vi "MainsubPanel.vi"() -> ()   [LabVIEW 2014]
doc: "Main\nThis is the main VI, and call via subpanel the other VI\n\nYou can click on the control and the selection on the menu.\n\nTo return in main subpanel press ESC.\n\n\nNicola Bavarone Bytelabs.it"
uses:
  SubPanel/SubPanelModule.lvlib
  MSQ_MessageQueues/Enqueue Message (Single).vi
  <vilib>/rvi/interface/nirviMethod/nirviMethod.xnode
  <vilib>/FPGAPlugInAG/Dynamic/niLvFpga_Reset_Dynamic.vi
  <vilib>/FPGAPlugInAG/Dynamic/niLvFpga_StartFifo_Dynamic.vi
  <vilib>/rvi/errors/niLvFpgaMergeErrorWithErrorCode.vi
  <vilib>/FPGAPlugInAG/Dynamic/niLvFpga_ConfigureFifo_Dynamic.vi
  <vilib>/FPGAPlugInAG/Dynamic/niLvFpga_Run_Dynamic.vi
  <vilib>/rvi/interface/nirviReadWriteControl/nirviReadWriteControl.xnode
  <vilib>/rvi/interface/Simulation/niFpgaSimulationCallBeginRW.vi
  <vilib>/rvi/errors/niLvFpgaAdjustHostInterfaceError.vi
  <vilib>/FPGAPlugInAG/Dynamic/niLvFpga_WriteFifo_Dynamic.vi
  <vilib>/rvi/interface/nirviCloseFPGA/nirviCloseFPGA.xnode
  <vilib>/FPGAPlugInAG/Dynamic/niLvFpga_Close_Dynamic.vi
  <vilib>/rvi/interface/nirviOpenFPGA/nirviOpenFPGA.xnode
  FPGA Bitfiles/LaserWaveMatrix_FPGATarget_LaserWaveFPGA_x7ByfWROQXI.lvbitx
  Fpga/FpgaMain.vi
panel:
  in  "NEW STRING":string="INSERISCI QUI LA TUA STRINGA"
  out "AO FIFO Empty":bool
  out "Empty Elements Remaining":u32
  out "# Loop":i32=83
  in  "Ton (ticks)":u32=40
  in  "Toff (ticks)":u32=40
  out "Elem act":u8
  in  "PRINT":bool
  out "Date":string
  out "Time":string
  # "EXTREME FM-X121"
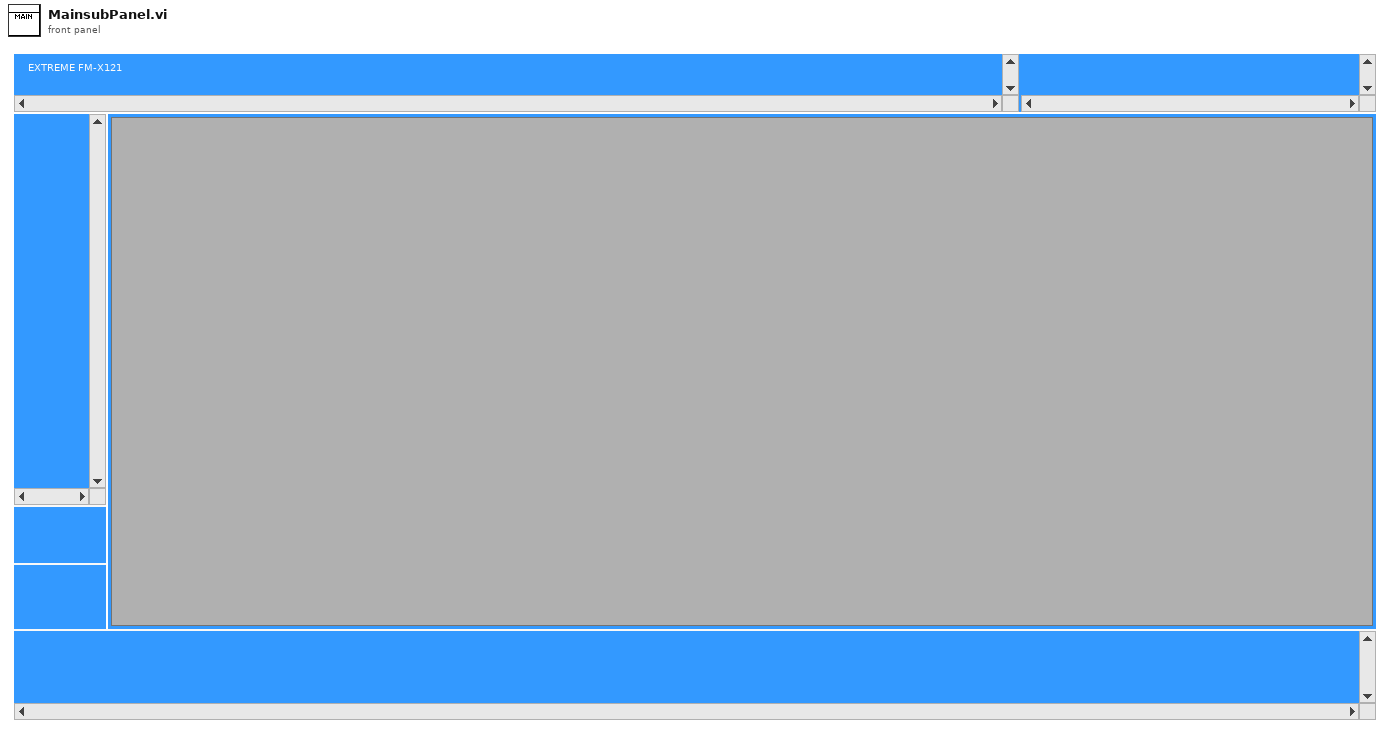
[diagram p1: front panel]
types:
  T1 = cluster{"Buffer_U64":u64[], "# Chart":i32, "BufferString":string[], "TotalStringBuff":i32, "over buffer":bool, "Ton (ticks)":u32, "Toff (ticks)":u32, "EmptyEl_Rem":u32}
  T2 = enum32{"invalid app kind", "Development System", "Run Time System", "Student Edition", "Embedded LabVIEW", "Evaluation", "Custom"}
  T3 = cluster{"UsrName":string, "UsrPsw":string, "UsrLevel":string}
  T4 = enum32{"Invalid", "Standard", "Closed", "Hidden", "Minimized", "Maximized"}
  T5 = typedef "eventvkey.ctl" = enum16{"ASCII", "Enter", "Return", "Shift", "Ctrl", "Alt", "Cmd", "Opt", "Caps", "NumLock", "Clear", "Break", "Up", "Down", "Left", "Right", "Insert", "Delete", "Home", "End", "PageUp", "PageDown", "Escape", "Help", "Pause", "ScrollLock", "F1", "F2", "F3", "F4", "F5", "F6", "F7", "F8", "F9", "F10", "F11", "F12", "F13", "F14", "F15", "F16", "F17", "F18", "F19", "F20", "F21", "F22", "F23", "F24", "Play", "VolumeUp", "VolumeDown", "Mute", "Two Byte Char"}
  T6 = enum32{"Bad", "Idle", "Run top level", "Running"}
  T7 = cluster{"Core":cluster{"Current VI Reference":refnum<vi>, "Close Panel on Exit?":bool}, "SubPanRefs":refnum<vi>[], "SubPanelsVis":string[], "SubP_VIsPathList":path[], "InsertedVIref":refnum<vi>, "Control Names":string[], "Values":variant[], "User":cluster{"UsrName":string, "UsrPsw":string, "UsrLevel":string}}
  T8 = cluster{"Current VI Reference":refnum<vi>, "Close Panel on Exit?":bool}
  T9 = typedef "Preset_Data.ctl" = cluster{"RS232config":T10, "USB_Config":T11, "PrintOffset":T12, "Aiming":T13, "Set Telnet TCPIP":T14}
  T10 = typedef "Rs232_Config.ctl" = cluster{"State":bool, "COM":string, "Baud Rate":i32, "Data Bit":i32, "Stop Bit":u16, "Parity":u16, "Flow Mode":u16}
  T11 = typedef "USB_Config.ctl" = cluster{"Status":bool, "COM":string}
  T12 = typedef "PrintOffset.ctl" = cluster{"PrintDelay":u32, "ForwardOffset":u32}
  T13 = typedef "Aiming.ctl" = cluster{"AimingBean":bool, "LaserTemperature":dbl, "SysTemperature":dbl}
  T14 = typedef "TCP_Config.ctl" = cluster{"State":bool, "IP ADDRESS":string, "Port":i32}
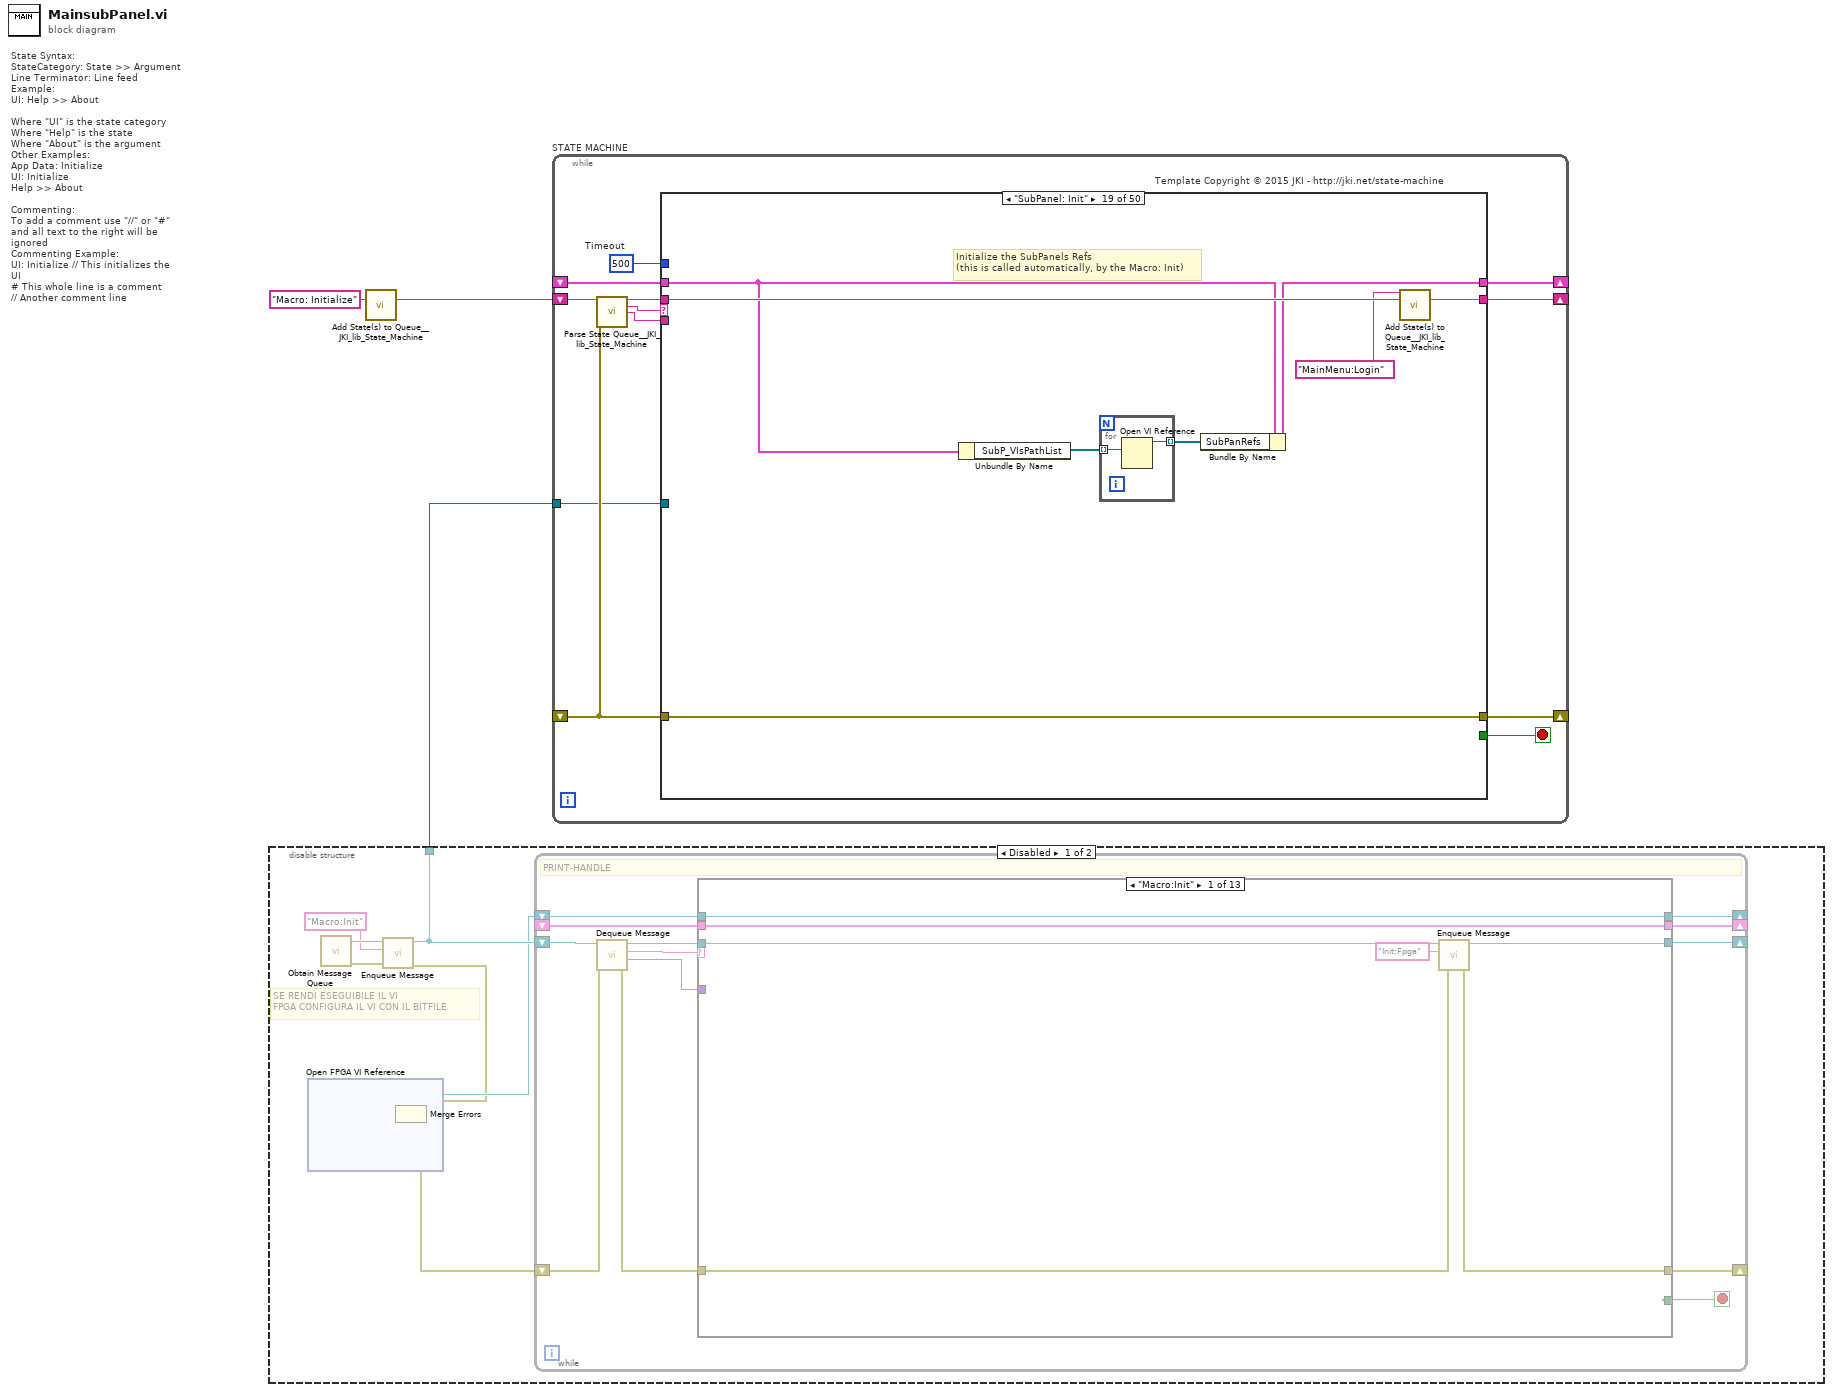
[diagram p0: block diagram]
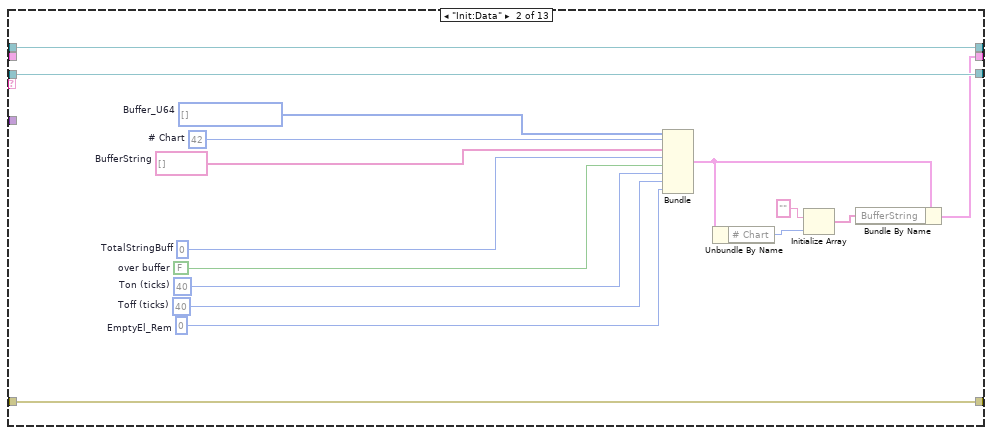
[diagram p2: hidden frame]
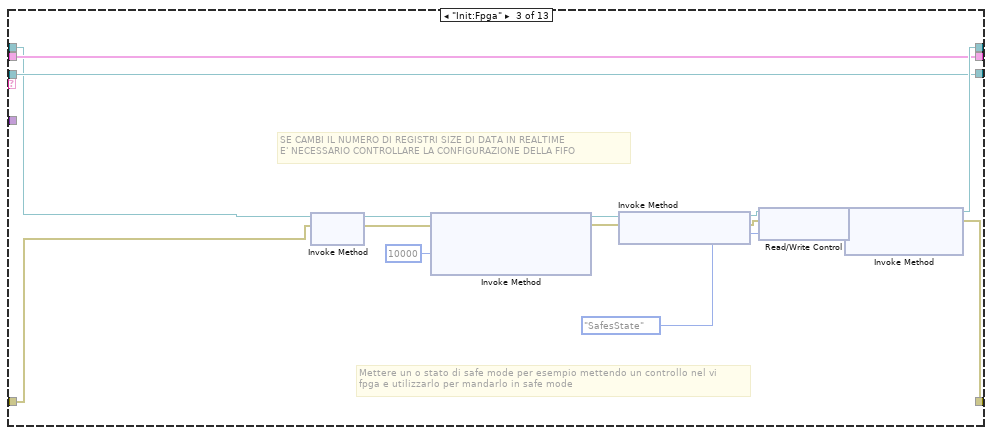
[diagram p3: hidden frame]
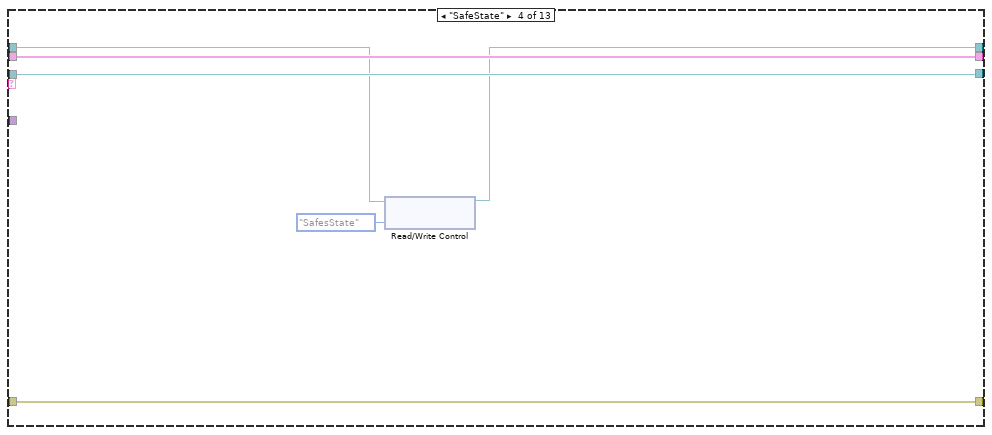
[diagram p4: hidden frame]
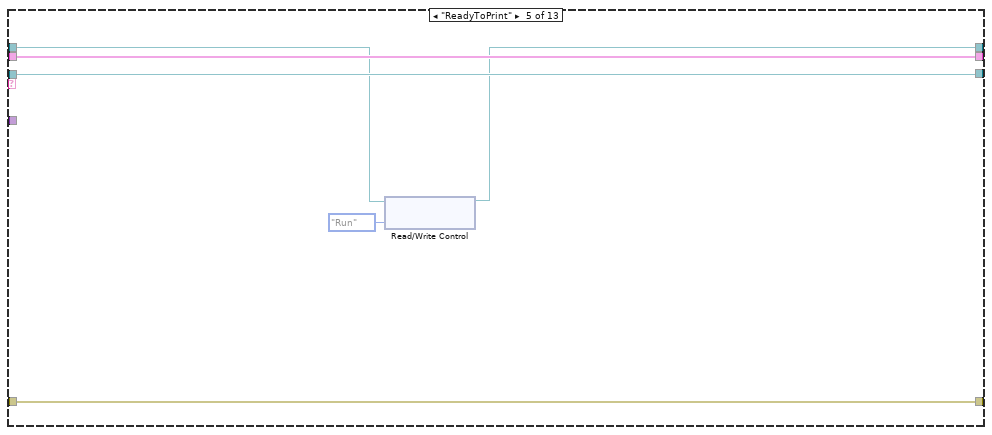
[diagram p5: hidden frame]
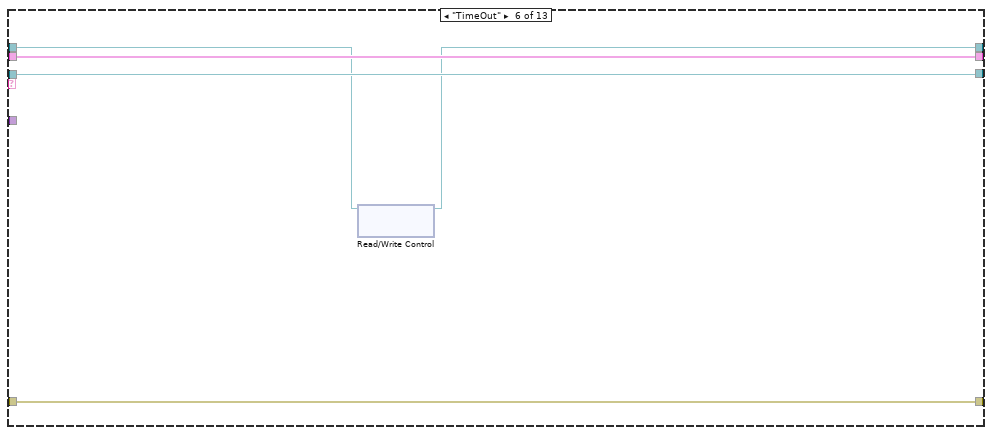
[diagram p6: hidden frame]
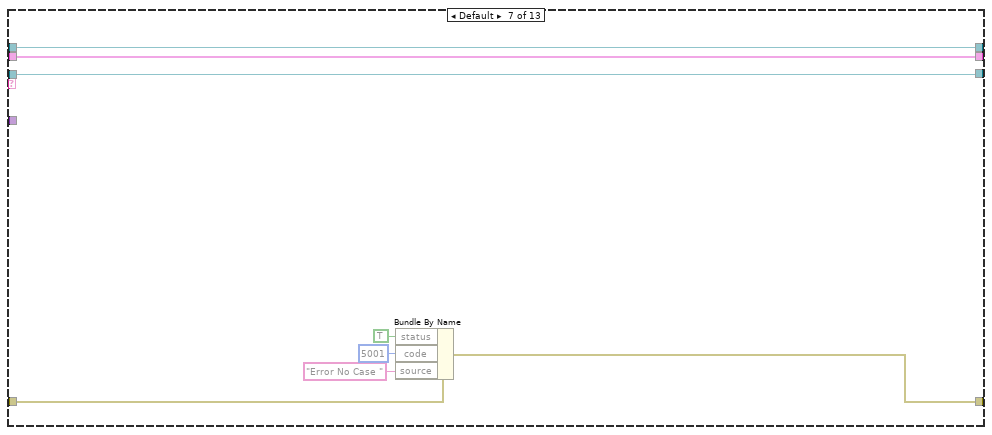
[diagram p7: hidden frame]
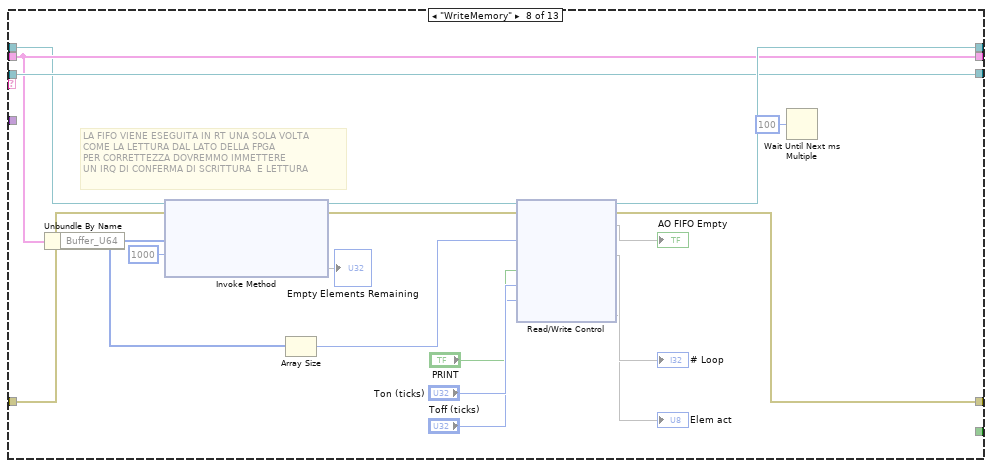
[diagram p8: hidden frame]
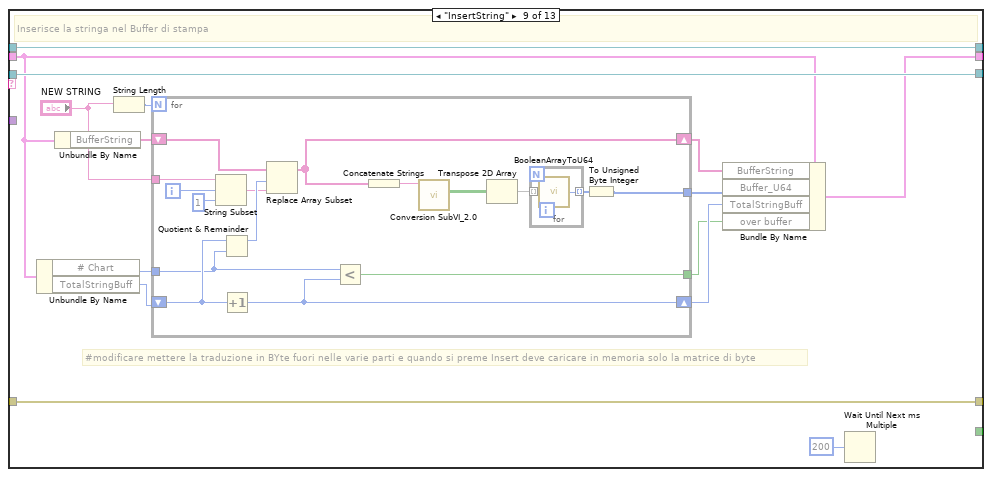
[diagram p9: hidden frame]
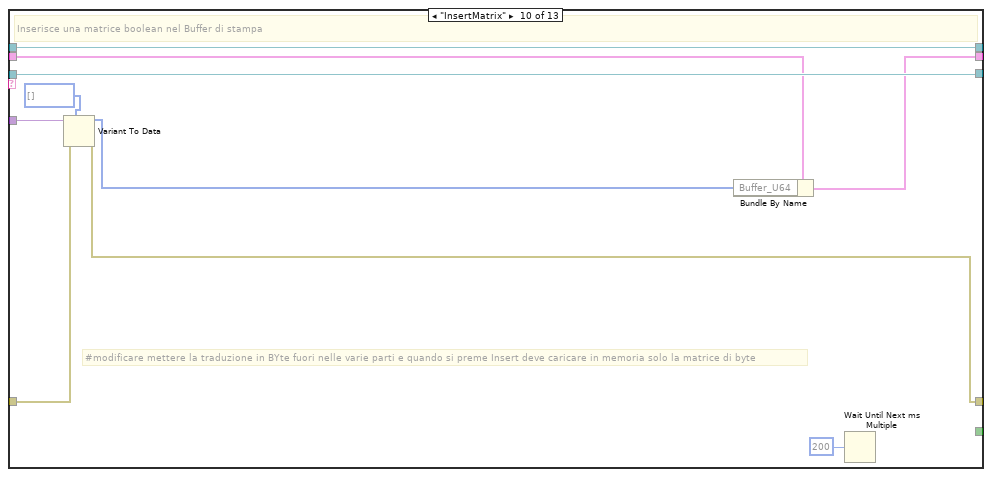
[diagram p10: hidden frame]
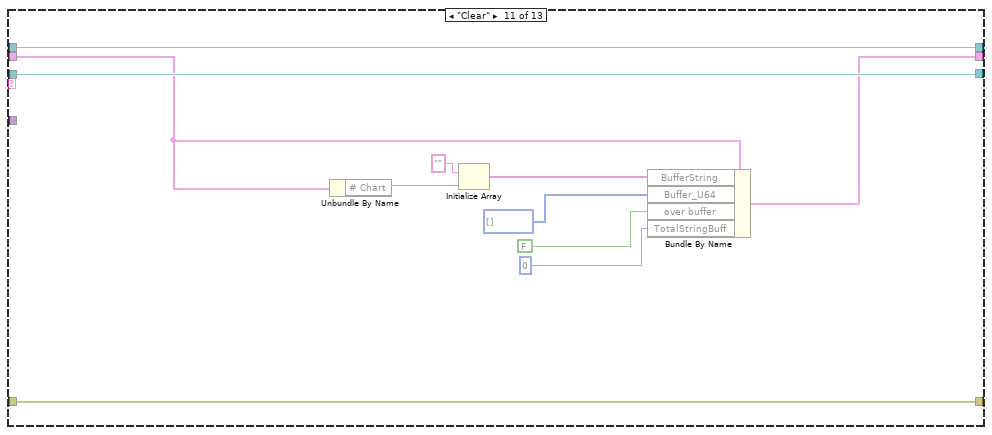
[diagram p11: hidden frame]
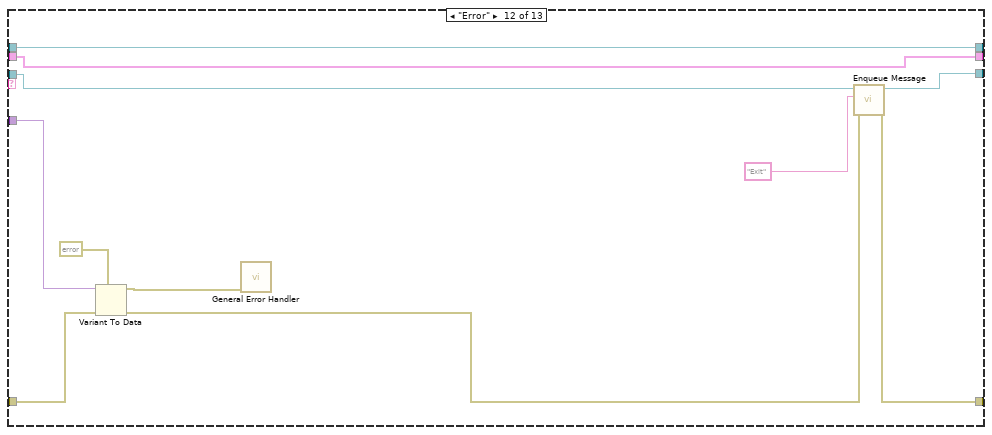
[diagram p12: hidden frame]
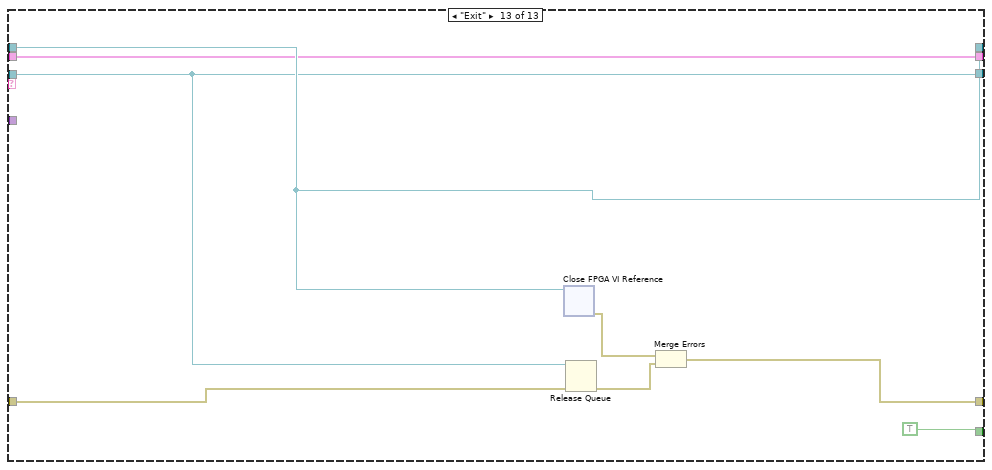
[diagram p13: hidden frame]
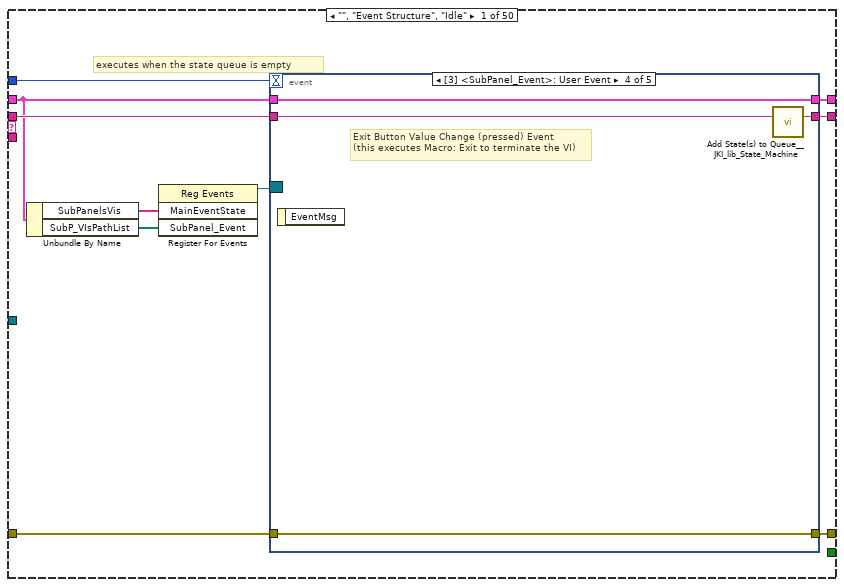
[diagram p15: hidden frame]
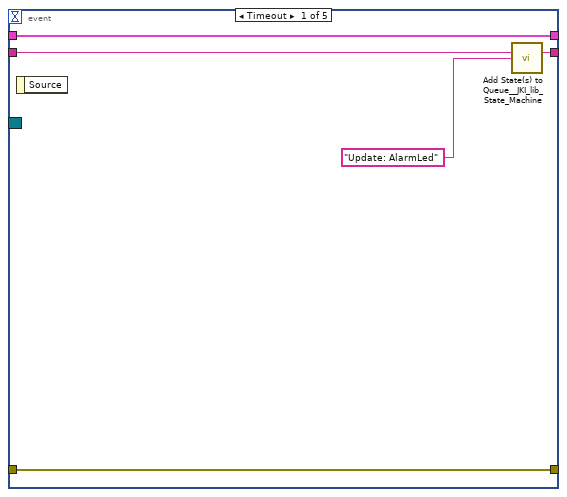
[diagram p16: hidden frame]
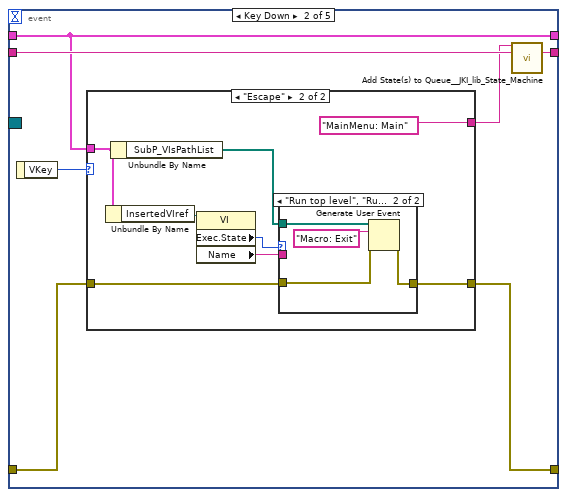
[diagram p17: hidden frame]
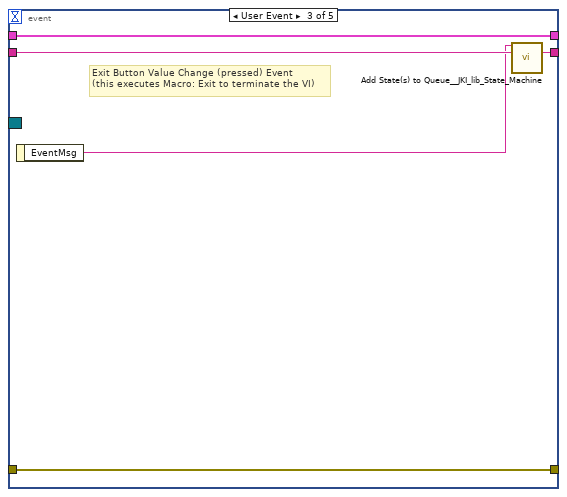
[diagram p20: hidden frame]
diagram:
  # "State Syntax:\nStateCategory: State >> Argument\nLine Terminator: Line feed\nExample:\nUI: Help >> About\n\nWhere \"UI\" is the state category\nWhere \"Help\" is the state\nWhere \"About\" is the argument\nOther Examples:\nApp Data: Initialize\nUI: Initialize\nHelp >> About\n\nCommenting:\nTo add a comment use \"//\" or \"#\" and all text to the right will be ignored\nCommenting Example:\nUI: Initialize // This initializes the UI\n# This whole line is a comment\n// Another comment line"
  n1 = disable-structure shown="Disabled" {
    disable-tunnel: [w8 _] -> w1
    frame Disabled {
      # "SE RENDI ESEGUIBILE IL VI \nFPGA CONFIGURA IL VI CON IL BITFILE"
      n2 = xnode "Open FPGA VI Reference"() -> ("FPGA VI Reference Out"=w7:refnum<k20>, "error out"=w6:errorcluster)  [unwired: 2 in]
      n3 = call "Obtain Message Queue.vi"() -> ("error out"=w10:errorcluster, "Message Queue"=w11:refnum<queue>)  [unwired: 10 in]
      n4 = call-poly "Enqueue Message.vi"("error in (no error)"=w10, "Message"="Macro:Init", "Message Queue"=w11) -> ("error out"=w4:errorcluster, "dup Message Queue"=w8:refnum<queue>)  [unwired: 7 in]
      n5 = Merge Errors(w4, w6) -> (w5:errorcluster)
      n6 = while {
        shift-right: [w22] -> _
        shift-left: w5 -> [w18]
        shift-right: [w23] -> _
        shift-left: w7 -> [w24]
        shift-right: [w20] -> _
        shift-left: w8 -> [w19]
        shift-right: [w12] -> _
        shift-left: _ -> [w13]
        stop <- w21 stop-if-true
        # "PRINT-HANDLE"
        n7 = call "Dequeue Message.vi"("error in (no error)"=w18, "Message Queue"=w19) -> ("error out"=w17:errorcluster, "Message Data"=w16:variant, "Message"=w15:string, "dup Message Queue"=w14:refnum<queue>)  [unwired: 6 in]
        n8 = case shown="\"Macro:Init\"" w15 {
          tunnel: w24 -> [w31 w46 w49 w66 w72 w77 w88 w89 w120 w149 w159 w168 w179]
          tunnel: w17 -> [w28 w47 w48 w69 w75 w80 w86 w105 w121 w141 w160 w167 w174]
          tunnel: [w27 w47 w57 w69 w75 w80 w87 w104 w121 w140 w160 w161 w173] -> w22
          tunnel: [w31 w46 w58 w65 w71 w76 w88 w102 w120 w149 w159 w168 w179] -> w23
          tunnel: w16 -> [_ _ _ _ _ _ _ _ _ w144 _ w171 _]
          tunnel: [_ _ _ _ _ _ _ _ _ _ _ _ TRUE] -> w21
          tunnel: [w29 w45 w56 w68 w74 w79 w82 w94 w119 w148 w158 w164 w175] -> w20
          tunnel: w14 -> [w30 w45 w56 w68 w74 w79 w82 w94 w119 w148 w158 w163 w175]
          tunnel: w13 -> [w25 _ w55 w67 w73 w78 w81 w91 w110 w145 w154 w166 w176]
          tunnel: [w25 w35 w55 w67 w73 w78 w81 w91 w116 w147 w155 w166 w176] -> w12
          frame "Macro:Init" {
            n9 = call-poly "Enqueue Message.vi"("error in (no error)"=w28, "Message"="Init:Fpga", "Message Queue"=w30) -> ("error out"=w27:errorcluster, "dup Message Queue"=w29:refnum<queue>)  [unwired: 7 in]
          }
          frame "Init:Data" {
            w39 = u32 0  # EmptyEl_Rem
            w40 = u32 40  # Toff (ticks)
            w41 = u32 40  # Ton (ticks)
            w42 = FALSE  # over buffer
            w43 = 0  # TotalStringBuff
            w36 = string[] []  # BufferString
            w37 = 42  # # Chart
            w44 = u64[] []  # Buffer_U64
            n10 = Bundle("Buffer_U64"=w44, "# Chart"=w37, "BufferString"=w36, "TotalStringBuff"=w43, "over buffer"=w42, "Ton (ticks)"=w41, "Toff (ticks)"=w40, "EmptyEl_Rem"=w39) -> (w32:T1)  [unwired: 1 in]
            n11 = Unbundle By Name(w32) -> ("# Chart"=w33:i32)
            n12 = Initialize Array("", w33) -> (w34:string[])
            n13 = Bundle By Name(cluster=w32, "BufferString"=w34) -> (w35:T1)
          }
          frame "Init:Fpga" {
            # "Mettere un o stato di safe mode per esempio mettendo un controllo nel vi\nfpga e utilizzarlo per mandarlo in safe mode"
            # "SE CAMBI IL NUMERO DI REGISTRI SIZE DI DATA IN REALTIME\nE' NECESSARIO CONTROLLARE LA CONFIGURAZIONE DELLA FIFO"
            n14 = xnode "Invoke Method"("FPGA VI Reference In"=w49, "error in"=w48) -> ("FPGA VI Reference Out"=w59:refnum<k20>, "error out"=w61:errorcluster)
            n15 = xnode "Invoke Method"("FPGA VI Reference In"=w59, "error in"=w61, "Requested Depth"=u32 10000) -> ("FPGA VI Reference Out"=w63:refnum<k20>, "error out"=w62:errorcluster)  [unwired: 1 out]
            n16 = xnode "Invoke Method"("FPGA VI Reference In"=w63, "error in"=w62) -> ("FPGA VI Reference Out"=w54:refnum<k20>, "error out"=w50:errorcluster)
            n17 = xnode "Read/Write Control"("FPGA VI Reference In"=w54, "error in"=w50, "FpgaOutState"=enum16{"SafesState", "Run"}."SafesState") -> ("FPGA VI Reference Out"=w52:refnum<k20>, "error out"=w51:errorcluster)
            n18 = xnode "Invoke Method"("FPGA VI Reference In"=w52, "error in"=w51) -> ("FPGA VI Reference Out"=w58:refnum<k20>, "error out"=w57:errorcluster)  [unwired: 1 in]
          }
          frame "SafeState" {
            n19 = xnode "Read/Write Control"("FPGA VI Reference In"=w66, "FpgaOutState"=enum16{"SafesState", "WriteMemory", "Run"}."SafesState") -> ("FPGA VI Reference Out"=w65:refnum<k20>)  [unwired: 1 in, 1 out]
          }
          frame "ReadyToPrint" {
            n20 = xnode "Read/Write Control"("FPGA VI Reference In"=w72, "FpgaOutState"=enum16{"SafesState", "WriteMemory", "Run"}."Run") -> ("FPGA VI Reference Out"=w71:refnum<k20>)  [unwired: 1 in, 1 out]
          }
          frame "TimeOut" {
            n21 = xnode "Read/Write Control"("FPGA VI Reference In"=w77) -> ("FPGA VI Reference Out"=w76:refnum<k20>)  [unwired: 1 in, 2 out]
          }
          frame Default {
            n22 = Bundle By Name(cluster=w86, "status"=TRUE, "code"=5001, "source"="Error No Case ") -> (w87:errorcluster)
          }
          frame "WriteMemory" {
            # "LA FIFO VIENE ESEGUITA IN RT UNA SOLA VOLTA\nCOME LA LETTURA DAL LATO DELLA FPGA\nPER CORRETTEZZA DOVREMMO IMMETTERE\nUN IRQ DI CONFERMA DI SCRITTURA  E LETTURA"
            n23 = Unbundle By Name(w91) -> ("Buffer_U64"=w90:u64[])
            n24 = xnode "Invoke Method"("FPGA VI Reference In"=w89, "error in"=w105, "Data"=w90, "Timeout (ms)"=1000) -> ("FPGA VI Reference Out"=w106:refnum<k20>, "error out"=w104:errorcluster, "Empty Elements Remaining"=→"Empty Elements Remaining")
            n25 = Array Size(array=w90) -> (size(s)=w100:i32)
            n26 = xnode "Read/Write Control"("FPGA VI Reference In"=w106, "size memory"=w100, "PRINT"="PRINT", "Ton (ticks)"="Ton (ticks)", "Toff (ticks)"="Toff (ticks)") -> ("FPGA VI Reference Out"=w102:refnum<k20>, "AO FIFO Empty"=→"AO FIFO Empty", "# Loop"=→"# Loop", "Elem act"=→"Elem act")  [unwired: 1 in, 1 out]
            n27 = Wait Until Next ms Multiple(millisecond multiple=u32 100) -> ()  [unwired: 1 out]
          }
          frame "InsertString" {
            # "#modificare mettere la traduzione in BYte fuori nelle varie parti e quando si preme Insert deve caricare in memoria solo la matrice di byte"
            # "Inserisce la stringa nel Buffer di stampa"
            n28 = Unbundle By Name(w110) -> ("# Chart"=w112:i32, "TotalStringBuff"=w108:i32)
            n29 = Unbundle By Name(w110) -> ("BufferString"=w111:string[])
            n30 = String Length(string="NEW STRING") -> (length=w118:i32)
            n31 = for {
              N: w118 -> [_]
              shift-right: [w131] -> w114
              shift-left: w111 -> [w137]
              shift-right: [w127] -> w109
              shift-left: w108 -> [w128]
              tunnel: "NEW STRING" -> [w133]
              tunnel: w112 -> [w126]
              tunnel: [w123] -> w115
              tunnel: [w122] -> w107
              i -> [w132]
              n32 = String Subset(string=w133, offset (0)=w132, length (rest)=1 ("length (rest)")) -> (substring=w134:string)
              n33 = Quotient & Remainder(x=w128, y=w126) -> (x-y*floor(x/y)=w136:i32)  [unwired: 1 out]
              n34 = Increment(x=w128) -> (x+1=w127:i32)
              n35 = Replace Array Subset "Replace Array Subset"(array=w137, new element=w134, index=w136) -> (w131:string[])
              n36 = Less?(x=w126, y=w127) -> (x < y?=w122:bool)
              n37 = Concatenate Strings "Concatenate Strings"(w131) -> (w129:string)
              n38 = call "Conversion SubVI_2.0.vi"("Input String"=w129) -> ("Boolean Array"=w125:bool[][])  [unwired: 9 in, 1 out]
              n39 = Transpose 2D Array(2D array=w125) -> (transposed array=w124:bool[][])
              n40 = for {
                tunnel: w124 -> [w139] mode=indexing
                tunnel: [w138] -> w130 mode=indexing
                n41 = call "BooleanArrayToU64.vi"("BooleanArray"=w139) -> ("Number(U64)"=w138:u64)  [unwired: 8 in]
              }
              n42 = To Unsigned Byte Integer(number=w130) -> (unsigned 8bit integer=w123:u8[])
            }
            n43 = Bundle By Name(cluster=w110, "BufferString"=w114, "Buffer_U64"=w115, "TotalStringBuff"=w109, "over buffer"=w107) -> (w116:T1)
            n44 = Wait Until Next ms Multiple(millisecond multiple=u32 200) -> ()  [unwired: 1 out]
          }
          frame "InsertMatrix" {
            # "#modificare mettere la traduzione in BYte fuori nelle varie parti e quando si preme Insert deve caricare in memoria solo la matrice di byte"
            # "Inserisce una matrice boolean nel Buffer di stampa"
            n45 = Variant To Data(error in=w141, type=u64[] [] ("Buffer_U64"), Variant=w144) -> (data=w142:u64[], error out=w140:errorcluster)
            n46 = Bundle By Name(cluster=w145, "Buffer_U64"=w142) -> (w147:T1)
            n47 = Wait Until Next ms Multiple(millisecond multiple=u32 200) -> ()  [unwired: 1 out]
          }
          frame "Clear" {
            n48 = Unbundle By Name(w154) -> ("# Chart"=w157:i32)
            n49 = Initialize Array("", w157) -> (w156:string[])
            n50 = Bundle By Name(cluster=w154, "BufferString"=w156, "Buffer_U64"=u8[] [] ("Array Num U8"), "over buffer"=FALSE, "TotalStringBuff"=0) -> (w155:T1)
          }
          frame "Error" {
            n51 = Variant To Data(error in=w167, type=errorcluster {"status"=FALSE, "code"=0, "source"=""} ("Error out"), Variant=w171) -> (data=w169:errorcluster, error out=w162:errorcluster)
            n52 = call <vilib>:"General Error Handler.vi"("error in (no error)"=w169) -> ()  [unwired: 10 in, 5 out]
            n53 = call-poly "Enqueue Message.vi"("error in (no error)"=w162, "Message"="Exit" ("Msg In"), "Message Queue"=w163) -> ("error out"=w161:errorcluster, "dup Message Queue"=w164:refnum<queue>)  [unwired: 7 in]
          }
          frame "Exit" {
            n54 = xnode "Close FPGA VI Reference"("FPGA VI Reference In"=w179) -> ("error out"=w177:errorcluster)  [unwired: 1 in]
            n55 = Release Queue(queue=w175, error in (no error)=w174) -> (error out=w172:errorcluster)  [unwired: 1 in, 2 out]
            n56 = Merge Errors(w177, w172) -> (w173:errorcluster)
          }
        }
      }
    }
    frame Enabled {
    }
  }
  n57 = call <vilib>:"Add State(s) to Queue__JKI_lib_State_Machine.vi"("State(s) in (\"\")"="Macro: Initialize") -> ("States Out"=w3:string)  [unwired: 14 in]
  n58 = while "STATE MACHINE" {
    shift-right: [w184] -> _
    shift-left: _ -> [w183]
    shift-right: [w187] -> _
    shift-left: _ -> [w181]
    shift-right: [w186] -> _
    shift-left: w3 -> [w188]
    tunnel: w1 -> [w180]
    stop <- w185 stop-if-true
    w182 = 500  # Timeout
    # "Template Copyright © 2015 JKI - http://jki.net/state-machine"
    n59 = call <vilib>:"Parse State Queue__JKI_lib_State_Machine.vi"("State Queue"=w188, "Error In (no error)"=w181) -> ("Remaining States"=w190:string, "Current State"=w191:string, "Arguments"=w189:string)  [unwired: 11 in]
    n60 = case shown="\"SubPanel: Init\"" w191 {
      selector: w191 -> [_ _ w247 _ _ _ _ _ _ _ _ _ _ _ _ _ _ _ _ _ _ _ _ _ _ _ _ _ _ _ _ _ _ _ _ _ _ _ _ _ _ _ _ _ _ _ _ _ w654 w661]
      tunnel: w190 -> [w201 w246 w251 w269 w275 w280 w284 w298 w304 w308 w312 w318 w333 w359 w364 w369 w379 w383 w391 w410 w414 w421 w428 w435 w442 w449 w456 w463 w470 w477 w481 w491 w501 w508 w518 w528 w538 w542 w550 w561 w577 w598 w602 w608 w619 w630 w642 w653 w655 w676]
      tunnel: w189 -> [_ _ _ _ _ _ _ _ _ _ _ w313 w327 _ _ _ _ _ _ w405 _ _ _ _ _ _ _ _ _ _ _ w489 w499 w506 w516 w526 _ _ _ w559 w564 w584 _ _ _ _ _ _ _ w670]
      tunnel: w183 -> [w193 w243 w249 w260 w272 w278 w281 _ w299 w305 w310 w316 w329 w356 w361 w366 w376 w380 w386 w396 w411 w418 w425 w432 w439 w446 w453 w460 w467 w474 w478 w488 w498 w502 w514 w524 w536 w539 w548 w552 w574 w596 w599 w606 w617 w628 w640 w650 w657 w663]
      tunnel: [w199 w244 w253 w266 errorcluster {"status"=FALSE, "code"=0, "source"=""} ("error out") w277 w282 w287 w300 w306 w309 w314 w330 w357 w362 w367 w377 w381 w389 w403 w412 w419 w426 w433 w440 w447 w454 w461 w468 w475 w479 w482 w493 w504 w510 w520 w535 w540 w543 w554 w575 w585 w600 w603 w614 w625 w637 w651 w658 w678] -> w187
      tunnel: w181 -> [w198 w244 w252 w266 w271 w277 w282 w286 w301 w306 w309 w315 w331 w357 w362 w367 w377 w381 w389 w404 w412 w419 w426 w433 w440 w447 w454 w461 w468 w475 w479 w486 w495 w505 w511 w521 w535 w540 w544 w555 w575 w586 w600 w604 w615 w626 w638 w651 w658 w678]
      tunnel: [w200 w245 w250 w268 w274 w279 w283 w297 w303 w307 w311 w317 w332 w358 w363 w368 w378 w382 w390 w409 w413 w420 w427 w434 w441 w448 w455 w462 w469 w476 w480 w490 w500 w507 w517 w527 w537 w541 w549 w560 w576 w597 w601 w607 w618 w629 w641 w652 w659 w679] -> w186
      tunnel: [_ _ _ _ _ TRUE _ _ _ _ _ _ _ _ _ _ _ _ _ _ _ _ _ _ _ _ _ _ _ _ _ _ _ _ _ _ _ _ _ _ _ _ _ _ _ _ _ _ _ _] -> w185
      tunnel: [w197 w243 w249 w267 w272 w278 w281 w296 w299 w305 w310 w316 w329 w356 w361 w366 w376 w380 w388 w401 w411 w418 w425 w432 w439 w446 w453 w460 w467 w474 w478 w484 w494 w502 w515 w525 w536 w539 w548 w551 w570 w592 w599 w606 w617 w628 w640 w650 w657 w660] -> w184
      tunnel: w182 -> [w196 _ _ _ _ _ _ _ _ _ _ _ _ _ _ _ _ _ _ _ _ _ _ _ _ _ _ _ _ _ _ _ _ _ _ _ _ _ _ _ _ _ _ _ _ _ _ _ _ _]
      tunnel: w180 -> [_ _ _ _ _ _ _ _ _ _ _ _ _ _ _ _ _ _ _ _ _ _ _ _ _ _ _ _ _ _ _ _ _ _ _ _ _ _ _ _ _ _ _ w605 w616 w627 w639 _ _ _]
      frame "", "Event Structure", "Idle" {
        # "executes when the state queue is empty"
        n61 = Unbundle By Name(w193) -> ("SubPanelsVis"=w194:string[], "SubP_VIsPathList"=w192:path[])
        n62 = register-events(w194, w192) -> (reference out=w195:refnum<event-registration>)  [unwired: 2 in, 1 out]
        n63 = event shown="[3] <SubPanel_Event>: User Event" {
          selector: w195 -> [_ _ _ _ _]
          dyn-events: _ -> [_ _ _ _ _]
          timeout: w196 -> [_ _ _ _ _]
          tunnel: w201 -> [w206 w213 w232 w236 w242]
          tunnel: [w205 w212 w231 w235 w241] -> w200
          tunnel: w193 -> [w203 w209 w229 w233 w239]
          tunnel: [w204 w207 w230 w234 w240] -> w199
          tunnel: w198 -> [w204 w208 w230 w234 w240]
          tunnel: [w203 w209 w229 w233 w239] -> w197
          event Timeout {
            n64 = event-data() -> ()  [unwired: 1 in, 1 out]
            n65 = call <vilib>:"Add State(s) to Queue__JKI_lib_State_Machine.vi"("State(s) in (\"\")"=w206, "State(s) at Back (\"\")"="Update: AlarmLed" ("State(s) at Back (\"\")")) -> ("States Out"=w205:string)  [unwired: 13 in]
          }
          event Key Down {
            n66 = event-data() -> ("VKey"=w211:T5)  [unwired: 1 in]
            n67 = case shown="\"Escape\"" w211 {
              tunnel: [_ "MainMenu: Main" ("State(s) in Front (\"\")")] -> w210
              tunnel: w209 -> [_ w218]
              tunnel: w208 -> [w214 w220]
              tunnel: [w214 w219] -> w207
              frame "ASCII", Default {
              }
              frame "Escape" {
                n68 = Unbundle By Name(w218) -> ("InsertedVIref"=w217:refnum<vi>)
                n69 = Unbundle By Name(w218) -> ("SubP_VIsPathList"=w221:path[])
                n70 = property class="VI"(reference=w217) -> ("Exec.State"=w216:T6, "Name"=w215:string)  [unwired: 1 in, 2 out]
                n71 = case shown="\"Run top level\", \"Running\"" w216 {
                  tunnel: w221 -> [_ w227]
                  tunnel: w220 -> [w223 w225]
                  tunnel: [w223 w224] -> w219
                  tunnel: w215 -> [_ _]
                  frame Default {
                  }
                  frame "Run top level", "Running" {
                    n72 = Generate User Event(user event=w227, event data cluster="Macro: Exit" ("event data"), error in=w225) -> (error out=w224:errorcluster)  [unwired: 1 in, 1 out]
                  }
                }
              }
            }
            n73 = call <vilib>:"Add State(s) to Queue__JKI_lib_State_Machine.vi"("State(s) in Front (\"\")"=w210, "State(s) in (\"\")"=w213) -> ("States Out"=w212:string)  [unwired: 13 in]
          }
          event User Event {
            # "Exit Button Value Change (pressed) Event\n(this executes Macro: Exit to terminate the VI)"
            n74 = event-data() -> ("EventMsg"=w228:string)  [unwired: 1 in]
            n75 = call <vilib>:"Add State(s) to Queue__JKI_lib_State_Machine.vi"("State(s) in Front (\"\")"=w228, "State(s) in (\"\")"=w232) -> ("States Out"=w231:string)  [unwired: 13 in]
          }
          event User Event {
            # "Exit Button Value Change (pressed) Event\n(this executes Macro: Exit to terminate the VI)"
            n76 = event-data() -> ()  [unwired: 1 in, 1 out]
            n77 = call <vilib>:"Add State(s) to Queue__JKI_lib_State_Machine.vi"("State(s) in (\"\")"=w236) -> ("States Out"=w235:string)  [unwired: 14 in]
          }
          event Panel Close? {
            # "Discard the event because we'll close the front panel ourselves in Macro: Exit"
            # "Close Panel button (pressed) Event\n(this executes Macro: Exit to terminate the VI)"
            n78 = event-data() -> ()  [unwired: 1 in, 1 out]
            n79 = event-data("Discard?"=TRUE) -> ()  [unwired: 1 in, 1 out]
            n80 = call <vilib>:"Add State(s) to Queue__JKI_lib_State_Machine.vi"("State(s) in Front (\"\")"="Macro: Exit", "State(s) in (\"\")"=w242) -> ("States Out"=w241:string)  [unwired: 13 in]
          }
        }
      }
      frame "---------- Core ----------" {
        # "Do not put any code in this frame.\n(it is a separator no-op)"
        n81 = call <vilib>:"Add State(s) to Queue__JKI_lib_State_Machine.vi"("State(s) in (\"\")"=w246) -> ("States Out"=w245:string)  [unwired: 14 in]
      }
      frame Default {
        w256 = 42 items=["No error", "Argument error", "Memory is full", "Out of zone", "End of file", "File already open", "Generic file I/O error", "File not found", "File permission error", "Disk is full", "Duplicate path", "Too many files open", "System feature not enabled", "Resource file not found", "Cannot add resource", "Resource not found", "Image not found", "Image memory error", "Pen does not exist", "Config type invalid", "Config token not found", "Config parse error", "Config memory error", "Bad external code format", "Bad external code offset", "External code not present", "Null window", "Destroy window error", "Null menu", "Print aborted", "Bad print record", "Print driver error", "Windows error during printing", "Memory error during printing", "Print dialog error", "Generic print error", "Invalid device refnum", "Device not found", "Device parameter error", "Device unit error", "Cannot open device", "Device call aborted", "Generic error", "Cancelled by user", "Object ID too low", "Object ID too high", "Object not in heap", "Unknown heap", "Unknown object (invalid DefProc)", "Unknown object (DefProc not in table)", "Message out of range", "Invalid (null) method", "Unknown message", "Manager call not supported", "Bad address", "Network operation in progress", "Network operation timed out", "Connection is busy", "Network attribute not supported", "Network error", "Address in use", "System out of memory", "Connection aborted", "Connection refused", "Not connected", "Already connected", "Connection closed", "Initialization error (interapplication manager)", "Bad occurrence", "Wait on unbound occurrence handler", "Occurrence queue overflow", "Datalog type conflict", "Unused", "Unrecognized type (interapplication manager)", "Memory corrupt", "Failed to make temporary DLL", "Old CIN version", "Drag socket not found", "Failed to load drop-object", "Failed to register OLE object", "Failed to release OLE object", "Format specifier type mismatch", "Unknown format specifier", "Too few format specifiers", "Too many format specifiers", "Scan failed", "Newer CIN version", "Error converting to variant", "Runtime menu error", "Password tampered", "Variant attribute not found", "Incompatible variant data type", "Event data is not available", "Event Store is not present", "Occurrence is not found", "Event Queue is not created", "Event info is not available", "Refnum passed is NULL", "Error retrieving Class GUID", "Error retrieving CoClass GUID", "Error retrieving TypeLib GUID.", "Bad built application magic bytes.", "Specific driver is different from the specific driver associated with the Logical Name.", "There is no session opened to the class driver.", "Max Error", "MAX - Error with config objects", "MAX - Error loading configuration", "MAX - Group not supported"]
        # "Current State"
        # "Do not delete, rename, or modify this frame.\n(this is used to capture unhandled states and typos)"
        # "Handle mistyped state name (developer tool)"
        n82 = Format Into String(format string="Software Exception: Unhandled State \"%s\"." ("message"), error in=w252, w247) -> (resulting string=w255:string, error out=w254:errorcluster)  [unwired: 1 in]
        n83 = call <vilib>:"Error Cluster From Error Code.vi"("show call chain? (False)"=TRUE, "error in (no error)"=w254, "error message (\"\")"=w255, "error code (0)"=w256) -> ("error out"=w253:errorcluster)  [unwired: 5 in]
        n84 = call <vilib>:"Add State(s) to Queue__JKI_lib_State_Machine.vi"("State(s) in (\"\")"=w251) -> ("States Out"=w250:string)  [unwired: 14 in]
      }
      frame "Initialize Core Data" {
        # "Do not delete, rename, or modify this frame.\n(this is used to determine panel behavior on exit)"
        # "originally closed?"
        # "exe?"
        # "If panel starts closed or is an EXE, then close it when we exit"
        n85 = property class="VI"() -> ("Front Panel.Open"=w265:bool)  [unwired: 2 in, 2 out]
        n86 = property class="App"() -> ("App.Kind"=w264:T2)  [unwired: 2 in, 2 out]
        n87 = control-ref of="Current VI Reference"() -> (w258:refnum<vi>)
        n88 = Not(x=w265) -> (.not. x?=w262:bool)
        n89 = Equal?(x=w264, y=T2."Run Time System" ("Application:Kind")) -> (x = y?=w261:bool)
        n90 = Or(x=w262, y=w261) -> (x .or. y?=w259:bool)
        n91 = Bundle By Name(cluster=w260, "Core.Current VI Reference"=w258, "Core.Close Panel on Exit?"=w259) -> (w267:T7)
        n92 = call <vilib>:"Add State(s) to Queue__JKI_lib_State_Machine.vi"("State(s) in (\"\")"=w269) -> ("States Out"=w268:string)  [unwired: 14 in]
      }
      frame "Error Handler" {
        # "Unhandled Error -- Display it"
        # "Handle any errors here.\nYou can also output any states to clean-up after errors occur"
        # "Clear error"
        n93 = call <vilib>:"General Error Handler.vi"("error in (no error)"=w271) -> ()  [unwired: 10 in, 5 out]
        n94 = call <vilib>:"Add State(s) to Queue__JKI_lib_State_Machine.vi"("State(s) in Front (\"\")"="/* Post Error States", "State(s) in (\"\")"=w275) -> ("States Out"=w274:string)  [unwired: 13 in]
      }
      frame "Exit" {
        # "Do not put any code in this frame.\n(No errors that occur here will be handled.)"
        n95 = call <vilib>:"Add State(s) to Queue__JKI_lib_State_Machine.vi"("State(s) in (\"\")"=w280) -> ("States Out"=w279:string)  [unwired: 14 in]
      }
      frame "---------- Data ----------" {
        # "Do not put any code in this frame.\n(It is a separator no-op. You can make a copy of this frame to create a new Data frame)"
        n96 = call <vilib>:"Add State(s) to Queue__JKI_lib_State_Machine.vi"("State(s) in (\"\")"=w284) -> ("States Out"=w283:string)  [unwired: 14 in]
      }
      frame "Data: Initialize" {
        w293 = refnum<vi> refnum  # InsertedVIref
        w294 = refnum<vi>[] []  # SubPanRefs
        w295 = T8 {"Current VI Reference"=refnum, "Close Panel on Exit?"=FALSE}  # Core
        # "do not delete - used by framework"
        # "Data names and types of shift register data are defined by this bundle."
        # "Initialize the shift-register data, here.\n(data names are defined by what you wire into the bundle function)"
        n97 = call "SubPanel_Path.vi"() -> ("SubPanelPath"=w292:path)  [unwired: 11 in]
        n98 = call "SubPanel_VIsList.vi"("error in (no error)"=w286, "SubPanelPath in"=w292) -> ("error out"=w287:errorcluster, "SubP_VIsPathList"=w290:path[], "SubPanelsVis"=w291:string[])  [unwired: 6 in, 1 out]
        n99 = Bundle("Core"=w295, "SubPanRefs"=w294, "SubPanelsVis"=w291, "SubP_VIsPathList"=w290, "InsertedVIref"=w293, "Control Names"=string[] [], "Values"=variant[] [], "User"=T3 {"UsrName"="", "UsrPsw"="", "UsrLevel"=""}) -> (w296:T7)  [unwired: 1 in]
        n100 = call <vilib>:"Add State(s) to Queue__JKI_lib_State_Machine.vi"("State(s) in (\"\")"=w298) -> ("States Out"=w297:string)  [unwired: 14 in]
      }
      frame "Data: Cleanup" {
        # "Cleanup any data and references, here.\n(this is called automatically, by the Macro: Exit)"
        n101 = Unbundle By Name(w299) -> ("Core.Current VI Reference"=w302:refnum<vi>)
        n102 = Close Reference(reference=w302, error in (no error)=w301) -> (error out=w300:errorcluster)
        n103 = call <vilib>:"Add State(s) to Queue__JKI_lib_State_Machine.vi"("State(s) in (\"\")"=w304) -> ("States Out"=w303:string)  [unwired: 14 in]
      }
      frame "---------- UI ----------" {
        # "Do not put any code in this frame.\n(It is a separator no-op. You can make a copy of this frame to create a new UI frame)"
        n104 = call <vilib>:"Add State(s) to Queue__JKI_lib_State_Machine.vi"("State(s) in (\"\")"=w308) -> ("States Out"=w307:string)  [unwired: 14 in]
      }
      frame "UI: Initialize" {
        # "Initialize the User Interface, here.\n(this is called automatically, by the Macro: Init)"
        n105 = call <vilib>:"Add State(s) to Queue__JKI_lib_State_Machine.vi"("State(s) in (\"\")"=w312) -> ("States Out"=w311:string)  [unwired: 14 in]
      }
      frame "UI: Cursor Set" {
        # "Argument"
        # "Set and Unset Cursor Busy.\n(Usage: \"UI: Cursor Set >> Busy|Idle\")"
        n106 = case shown="\"Idle\", Default" w313 {
          tunnel: w315 -> [w320 w324]
          tunnel: [w319 w323] -> w314
          frame "Idle", Default {
            n107 = disable-structure shown="Disabled" {
              disable-tunnel: w320 -> [w322 _]
              disable-tunnel: [w321 _] -> w319
              frame Disabled {
                n108 = call <vilib>:"Unset Busy.vi"("error in (no error)"=w322) -> ("error out"=w321:errorcluster)  [unwired: 10 in]
              }
              frame Enabled {
              }
            }
          }
          frame "Busy" {
            n109 = disable-structure shown="Disabled" {
              disable-tunnel: w324 -> [w326 _]
              disable-tunnel: [w325 _] -> w323
              frame Disabled {
                n110 = call <vilib>:"Set Busy.vi"("error in (no error)"=w326) -> ("error out"=w325:errorcluster)  [unwired: 9 in, 1 out]
              }
              frame Enabled {
              }
            }
          }
        }
        n111 = call <vilib>:"Add State(s) to Queue__JKI_lib_State_Machine.vi"("State(s) in (\"\")"=w318) -> ("States Out"=w317:string)  [unwired: 14 in]
      }
      frame "UI: Front Panel State" {
        # "Argument"
        # "Set Front Panel Open or Closed\n(Usage: \"UI: Front Panel State >> Open|Close\")"
        n112 = Unbundle By Name(w329) -> ("Core.Current VI Reference"=w328:refnum<vi>)
        n113 = case shown="\"Close\"" w327 {
          tunnel: w331 -> [w337 w350]
          tunnel: [w339 w351] -> w330
          tunnel: w328 -> [w338 w348]
          frame "Open", Default {
            n114 = property class="VI"(reference=w338, error in=w337) -> (reference out=w335:refnum<vi>, error out=w336:errorcluster, "Front Panel.Open"=w334:bool)
            n115 = case shown="False" w334 {
              tunnel: [w342 w345] -> w339
              tunnel: w336 -> [w341 w345]
              tunnel: w335 -> [w340 _]
              frame False {
                n116 = invoke class="VI" method="FP.Open"(reference=w340, error in=w341, "Activate"=TRUE, "State"=T4."Standard") -> (error out=w342:errorcluster)  [unwired: 1 in, 4 out]
              }
              frame True {
              }
            }
          }
          frame "Close" {
            n117 = property class="VI"(reference=w348, error in=w350) -> (reference out=w347:refnum<vi>, error out=w349:errorcluster, "Front Panel.Open"=w346:bool)
            n118 = case shown="True" w346 {
              tunnel: [w352 w355] -> w351
              tunnel: w349 -> [w352 w354]
              tunnel: w347 -> [_ w353]
              frame False {
              }
              frame True {
                n119 = invoke class="VI" method="FP.Close"(reference=w353, error in=w354) -> (error out=w355:errorcluster)  [unwired: 1 in, 2 out]
              }
            }
          }
        }
        n120 = call <vilib>:"Add State(s) to Queue__JKI_lib_State_Machine.vi"("State(s) in (\"\")"=w333) -> ("States Out"=w332:string)  [unwired: 14 in]
      }
      frame "---------- Macro ----------" {
        # "Do not put any code in this frame.\n(It is a separator no-op. You can make a copy of this frame to create a new Macro frame)"
        n121 = call <vilib>:"Add State(s) to Queue__JKI_lib_State_Machine.vi"("State(s) in (\"\")"=w359) -> ("States Out"=w358:string)  [unwired: 14 in]
      }
      frame "Macro: Initialize" {
        w360 = "Data: Initialize\nInitialize Core Data\nUI: Initialize\nUI: Front Panel State >> Open\nSubPanel: Init"  # Data: Initialize Initialize Core Data UI: Initialize UI: Front Panel State >> Open SubPanel: Init
        # "Initialization Macro\n(This is called once, when the VI starts)"
        n122 = call <vilib>:"Add State(s) to Queue__JKI_lib_State_Machine.vi"("State(s) in Front (\"\")"=w360, "State(s) in (\"\")"=w364) -> ("States Out"=w363:string)  [unwired: 13 in]
      }
      frame "Macro: Timeout" {
        # "Timeout Macro\n(This is called on Timeout event.)"
        n123 = call <vilib>:"Add State(s) to Queue__JKI_lib_State_Machine.vi"("State(s) in Front (\"\")"="Update: DateTime\nUpdate: AlarmLed", "State(s) in (\"\")"=w369) -> ("States Out"=w368:string)  [unwired: 13 in]
      }
      frame "Macro: Exit" {
        # "Exit Macro\n(This is called once, when the VI exits)"
        n124 = Unbundle By Name(w376) -> ("Core.Close Panel on Exit?"=w375:bool)
        n125 = Select(t="UI: Front Panel State >> Close", s=w375, f="") -> (s? t:f=w372:string)
        n126 = call <vilib>:"Add State(s) to Queue__JKI_lib_State_Machine.vi"("State(s) in (\"\")"=w372, "State(s) at Back (\"\")"="Data: Cleanup\nExit") -> ("States Out"=w370:string)  [unwired: 13 in]
        n127 = call <vilib>:"Add State(s) to Queue__JKI_lib_State_Machine.vi"("State(s) in Front (\"\")"=w370, "State(s) in (\"\")"=w379) -> ("States Out"=w378:string)  [unwired: 13 in]
      }
      frame "---------- SubPanel ----------" {
        # "Template Separator\n(You can make a copy of, or modify, this frame)"
        n128 = call <vilib>:"Add State(s) to Queue__JKI_lib_State_Machine.vi"("State(s) in (\"\")"=w383) -> ("States Out"=w382:string)  [unwired: 14 in]
      }
      frame "SubPanel: Init" {
        # "Initialize the SubPanels Refs\n(this is called automatically, by the Macro: Init)"
        n129 = Unbundle By Name(w386) -> ("SubP_VIsPathList"=w384:path[])
        n130 = for {
          tunnel: w384 -> [w392] mode=indexing
          tunnel: [w393] -> w387 mode=indexing
          n131 = Open VI Reference(vi path=w392) -> (vi reference=w393:refnum<vi>)  [unwired: 5 in, 1 out]
        }
        n132 = Bundle By Name(cluster=w386, "SubPanRefs"=w387) -> (w388:T7)
        n133 = call <vilib>:"Add State(s) to Queue__JKI_lib_State_Machine.vi"("State(s) in Front (\"\")"="MainMenu:Login" ("State(s) in Front (\"\")"), "State(s) in (\"\")"=w391) -> ("States Out"=w390:string)  [unwired: 13 in]
      }
      frame "SubPanel: Load" {
        # "Importante:\nCAncello i control names\nper evitare di chiamare per altri subVIS"
        # "Load VI on the SubPanel\n(Load the VI on subpanel)"
        n134 = Unbundle By Name(w396) -> ("SubPanelsVis"=w406:string[])
        n135 = Unbundle By Name(w396) -> ("SubPanRefs"=w407:refnum<vi>[])
        n136 = control-ref of="Sub Panel"() -> (w408:refnum<vi>)
        n137 = call "SubPanel_InsertVI.vi"("SubPanVI_Names"=w406, "error in (no error)"=w404, "SubPanRefs"=w407, "InsertVI_Name"=w405, "SubPanel in"=w408) -> ("error out"=w402:errorcluster, "InsertedVI"=w400:refnum<vi>)  [unwired: 5 in]
        n138 = Unbundle By Name(w396) -> ("Control Names"=w397:string[], "Values"=w398:variant[])
        n139 = call "SubPanel_RunVI_Parameter.vi"("error in (no error)"=w402, "Values"=w398, "Control Names"=w397, "VIref in"=w400) -> ("error out"=w403:errorcluster, "VIref out"=w399:refnum<vi>)  [unwired: 6 in]
        n140 = Bundle By Name(cluster=w396, "InsertedVIref"=w399, "Control Names"=string[] [], "Values"=variant[] []) -> (w401:T7)
        n141 = call <vilib>:"Add State(s) to Queue__JKI_lib_State_Machine.vi"("State(s) in (\"\")"=w410) -> ("States Out"=w409:string)  [unwired: 14 in]
      }
      frame "---------- Main Menu ----------" {
        # "o not put any code in this frame.\n(It is a separator no-op. You can make a copy of this frame to create a new UI frame)\n(You can make a copy of, or modify, this frame)"
        n142 = call <vilib>:"Add State(s) to Queue__JKI_lib_State_Machine.vi"("State(s) in (\"\")"=w414) -> ("States Out"=w413:string)  [unwired: 14 in]
      }
      frame "MainMenu: Main" {
        # "Call Setup Service from Main Menu dynamic vi\n(Il MAin Menu manda un evento che contiene una stringa di chiamata a questo case)\n(You can make a copy of, or modify, this frame)"
        n143 = call <vilib>:"Build State String with Arguments__JKI_lib_State_Machine.vi"("Arguments (\"\")"="MainMenu.vi" ("Arguments (\"\")"), "State"="SubPanel: Load" ("State(s) in Front (\"\")")) -> ("State with Arguments"=w415:string)  [unwired: 4 in]
        n144 = call <vilib>:"Add State(s) to Queue__JKI_lib_State_Machine.vi"("State(s) in Front (\"\")"=w415, "State(s) in (\"\")"=w421) -> ("States Out"=w420:string)  [unwired: 13 in]
      }
      frame "MainMenu:Login" {
        # "Call Setup Service from Main Menu dynamic vi\n(Il MAin Menu manda un evento che contiene una stringa di chiamata a questo case)\n(You can make a copy of, or modify, this frame)"
        n145 = call <vilib>:"Build State String with Arguments__JKI_lib_State_Machine.vi"("Arguments (\"\")"="Login.vi" ("Arguments (\"\")"), "State"="SubPanel: Load" ("State(s) in Front (\"\")")) -> ("State with Arguments"=w422:string)  [unwired: 4 in]
        n146 = call <vilib>:"Add State(s) to Queue__JKI_lib_State_Machine.vi"("State(s) in Front (\"\")"=w422, "State(s) in (\"\")"=w428) -> ("States Out"=w427:string)  [unwired: 13 in]
      }
      frame "MainMenu: SETUP-SERVICE" {
        # "Call Setup Service from Main Menu dynamic vi\n(Il MAin Menu manda un evento che contiene una stringa di chiamata a questo case)\n(You can make a copy of, or modify, this frame)"
        n147 = call <vilib>:"Build State String with Arguments__JKI_lib_State_Machine.vi"("Arguments (\"\")"="SETUP-SERVICE.vi" ("Arguments (\"\")"), "State"="SubPanel: Load" ("State(s) in Front (\"\")")) -> ("State with Arguments"=w429:string)  [unwired: 4 in]
        n148 = call <vilib>:"Add State(s) to Queue__JKI_lib_State_Machine.vi"("State(s) in Front (\"\")"=w429, "State(s) in (\"\")"=w435) -> ("States Out"=w434:string)  [unwired: 13 in]
      }
      frame "MainMenu: SETUP LIST" {
        # "Call Setup Service from Main Menu dynamic vi\n(Il MAin Menu manda un evento che contiene una stringa di chiamata a questo case)\n(You can make a copy of, or modify, this frame)"
        n149 = call <vilib>:"Build State String with Arguments__JKI_lib_State_Machine.vi"("Arguments (\"\")"="SetupList.vi" ("Arguments (\"\")"), "State"="SubPanel: Load" ("State(s) in Front (\"\")")) -> ("State with Arguments"=w436:string)  [unwired: 4 in]
        n150 = call <vilib>:"Add State(s) to Queue__JKI_lib_State_Machine.vi"("State(s) in Front (\"\")"=w436, "State(s) in (\"\")"=w442) -> ("States Out"=w441:string)  [unwired: 13 in]
      }
      frame "MainMenu: EDITOR" {
        # "Call Setup Service from Main Menu dynamic vi\n(Il MAin Menu manda un evento che contiene una stringa di chiamata a questo case)\n(You can make a copy of, or modify, this frame)"
        n151 = call <vilib>:"Build State String with Arguments__JKI_lib_State_Machine.vi"("Arguments (\"\")"="MessageEditor.vi" ("Arguments (\"\")"), "State"="SubPanel: Load" ("State(s) in Front (\"\")")) -> ("State with Arguments"=w443:string)  [unwired: 4 in]
        n152 = call <vilib>:"Add State(s) to Queue__JKI_lib_State_Machine.vi"("State(s) in Front (\"\")"=w443, "State(s) in (\"\")"=w449) -> ("States Out"=w448:string)  [unwired: 13 in]
      }
      frame "MainMenu: COMMUNICATION" {
        # "Call Setup Service from Main Menu dynamic vi\n(Il MAin Menu manda un evento che contiene una stringa di chiamata a questo case)\n(You can make a copy of, or modify, this frame)"
        n153 = call <vilib>:"Build State String with Arguments__JKI_lib_State_Machine.vi"("Arguments (\"\")"="Communication.vi" ("Arguments (\"\")"), "State"="SubPanel: Load" ("State(s) in Front (\"\")")) -> ("State with Arguments"=w450:string)  [unwired: 4 in]
        n154 = call <vilib>:"Add State(s) to Queue__JKI_lib_State_Machine.vi"("State(s) in Front (\"\")"=w450, "State(s) in (\"\")"=w456) -> ("States Out"=w455:string)  [unwired: 13 in]
      }
      frame "MainMenu: DATE & TIME" {
        # "Call Setup Service from Main Menu dynamic vi\n(Il MAin Menu manda un evento che contiene una stringa di chiamata a questo case)\n(You can make a copy of, or modify, this frame)"
        n155 = call <vilib>:"Build State String with Arguments__JKI_lib_State_Machine.vi"("Arguments (\"\")"="DateTime.vi" ("Arguments (\"\")"), "State"="SubPanel: Load" ("State(s) in Front (\"\")")) -> ("State with Arguments"=w457:string)  [unwired: 4 in]
        n156 = call <vilib>:"Add State(s) to Queue__JKI_lib_State_Machine.vi"("State(s) in Front (\"\")"=w457, "State(s) in (\"\")"=w463) -> ("States Out"=w462:string)  [unwired: 13 in]
      }
      frame "MainMenu: LINE SPEED & CHAR LENGHT" {
        # "Call Setup Service from Main Menu dynamic vi\n(Il MAin Menu manda un evento che contiene una stringa di chiamata a questo case)\n(You can make a copy of, or modify, this frame)"
        n157 = call <vilib>:"Build State String with Arguments__JKI_lib_State_Machine.vi"("Arguments (\"\")"="PrintOffset.vi" ("Arguments (\"\")"), "State"="SubPanel: Load" ("State(s) in Front (\"\")")) -> ("State with Arguments"=w464:string)  [unwired: 4 in]
        n158 = call <vilib>:"Add State(s) to Queue__JKI_lib_State_Machine.vi"("State(s) in Front (\"\")"=w464, "State(s) in (\"\")"=w470) -> ("States Out"=w469:string)  [unwired: 13 in]
      }
      frame "MainMenu: Service" {
        # "Call Setup Service from Main Menu dynamic vi\n(Il MAin Menu manda un evento che contiene una stringa di chiamata a questo case)\n(You can make a copy of, or modify, this frame)"
        n159 = call <vilib>:"Build State String with Arguments__JKI_lib_State_Machine.vi"("Arguments (\"\")"="SystemService.vi" ("Arguments (\"\")"), "State"="SubPanel: Load" ("State(s) in Front (\"\")")) -> ("State with Arguments"=w471:string)  [unwired: 4 in]
        n160 = call <vilib>:"Add State(s) to Queue__JKI_lib_State_Machine.vi"("State(s) in Front (\"\")"=w471, "State(s) in (\"\")"=w477) -> ("States Out"=w476:string)  [unwired: 13 in]
      }
      frame "-------------Update-------------" {
        # "o not put any code in this frame.\n(It is a separator no-op. You can make a copy of this frame to create a new UI frame)\n(You can make a copy of, or modify, this frame)"
        n161 = call <vilib>:"Add State(s) to Queue__JKI_lib_State_Machine.vi"("State(s) in (\"\")"=w481) -> ("States Out"=w480:string)  [unwired: 14 in]
      }
      frame "Update: RS232config" {
        # "Aggiorno la RS232\n(aggiorna la RS232)"
        n162 = Unbundle By Name(w488) -> ("RS232config"=w487)
        n163 = Unflatten From String(type=w487, binary string=w489, error in (no error)=w486) -> (value=w485, error out=w482:errorcluster)  [unwired: 2 in, 1 out]
        n164 = Bundle By Name(cluster=w488, "RS232config"=w485) -> (w484:T7)
        n165 = call <vilib>:"Add State(s) to Queue__JKI_lib_State_Machine.vi"("State(s) in (\"\")"=w491, "State(s) at Back (\"\")"="Preset:UpdatePresentPreset" ("State(s) at Back (\"\")")) -> ("States Out"=w490:string)  [unwired: 13 in]
      }
      frame "Update: PrintOffset" {
        # "o not put any code in this frame.\n(It is a separator no-op. You can make a copy of this frame to create a new UI frame)\n(You can make a copy of, or modify, this frame)"
        n166 = Unbundle By Name(w498) -> ("PrintOffset"=w497)
        n167 = Unflatten From String(type=w497, binary string=w499, error in (no error)=w495) -> (value=w496, error out=w493:errorcluster)  [unwired: 2 in, 1 out]
        n168 = Bundle By Name(cluster=w498, "PrintOffset"=w496) -> (w494:T7)
        n169 = call <vilib>:"Add State(s) to Queue__JKI_lib_State_Machine.vi"("State(s) in (\"\")"=w501, "State(s) at Back (\"\")"="Preset:UpdatePresentPreset" ("State(s) at Back (\"\")")) -> ("States Out"=w500:string)  [unwired: 13 in]
      }
      frame "Update: Power" {
        w503 = u8 0  # Power
        # "Aggiorno la Potenza del sensore\n(It is a separator no-op. You can make a copy of this frame to create a new UI frame)\n(You can make a copy of, or modify, this frame)"
        n170 = Unflatten From String(type=w503, binary string=w506, error in (no error)=w505) -> (error out=w504:errorcluster)  [unwired: 2 in, 2 out]
        n171 = call <vilib>:"Add State(s) to Queue__JKI_lib_State_Machine.vi"("State(s) in (\"\")"=w508) -> ("States Out"=w507:string)  [unwired: 14 in]
      }
      frame "Update: USBconfig" {
        # "o not put any code in this frame.\n(It is a separator no-op. You can make a copy of this frame to create a new UI frame)\n(You can make a copy of, or modify, this frame)"
        n172 = Unbundle By Name(w514) -> ("USB_Config"=w513)
        n173 = Unflatten From String(type=w513, binary string=w516, error in (no error)=w511) -> (value=w512, error out=w510:errorcluster)  [unwired: 2 in, 1 out]
        n174 = Bundle By Name(cluster=w514, "USB_Config"=w512) -> (w515:T7)
        n175 = call <vilib>:"Add State(s) to Queue__JKI_lib_State_Machine.vi"("State(s) in (\"\")"=w518, "State(s) at Back (\"\")"="Preset:UpdatePresentPreset" ("State(s) at Back (\"\")")) -> ("States Out"=w517:string)  [unwired: 13 in]
      }
      frame "Update: Aiming" {
        # "o not put any code in this frame.\n(It is a separator no-op. You can make a copy of this frame to create a new UI frame)\n(You can make a copy of, or modify, this frame)"
        n176 = Unbundle By Name(w524) -> ("Aiming"=w523)
        n177 = Unflatten From String(type=w523, binary string=w526, error in (no error)=w521) -> (value=w522, error out=w520:errorcluster)  [unwired: 2 in, 1 out]
        n178 = Bundle By Name(cluster=w524, "Aiming"=w522) -> (w525:T7)
        n179 = call <vilib>:"Add State(s) to Queue__JKI_lib_State_Machine.vi"("State(s) in (\"\")"=w528, "State(s) at Back (\"\")"="Preset:UpdatePresentPreset" ("State(s) at Back (\"\")")) -> ("States Out"=w527:string)  [unwired: 13 in]
      }
      frame "Update: DateTime" {
        # "Aggiornamento Data e ora\n(It is a separator no-op. You can make a copy of this frame to create a new UI frame)\n(You can make a copy of, or modify, this frame)"
        n180 = Get Date/Time In Seconds() -> (seconds since 1Jan1904=w532:timestamp)
        n181 = Get Date/Time In Seconds() -> (seconds since 1Jan1904=w534:timestamp)
        n182 = Format Date/Time String(time format string (%c)="%H:%M:%S" ("FormatTime"), seconds (now)=w532) -> (date/time string=→"Time":string)  [unwired: 1 in]
        n183 = Format Date/Time String(time format string (%c)="%d-%m-%4Y" ("FORMAT"), seconds (now)=w534) -> (date/time string=→"Date":string)  [unwired: 1 in]
        n184 = call <vilib>:"Add State(s) to Queue__JKI_lib_State_Machine.vi"("State(s) in (\"\")"=w538) -> ("States Out"=w537:string)  [unwired: 14 in]
      }
      frame "-----------Preset------------" {
        # "o not put any code in this frame.\n(It is a separator no-op. You can make a copy of this frame to create a new UI frame)\n(You can make a copy of, or modify, this frame)"
        n185 = call <vilib>:"Add State(s) to Queue__JKI_lib_State_Machine.vi"("State(s) in (\"\")"=w542) -> ("States Out"=w541:string)  [unwired: 14 in]
      }
      frame "Preset:UpdatePresentPreset" {
        # "Aggiorna il preset attuale\n(Tutte le volte che un preset viene modificato utilizzare questa funzione per aggiornare l'xml del preset attivo)"
        n186 = Unbundle By Name(w548) -> ("Control Names"=w547:string[], "Values"=w546:variant[])
        n187 = call "SettingDataXML.vi"("SettingDataXmlPath"=w547, "error IO"=w544, "Actions"=enum16{"Init", "Read", "Write"}."Write", "Setting In"=w546) -> ("error out"=w543:errorcluster)  [unwired: 6 in, 1 out]
        n188 = call <vilib>:"Add State(s) to Queue__JKI_lib_State_Machine.vi"("State(s) in (\"\")"=w550) -> ("States Out"=w549:string)  [unwired: 14 in]
      }
      frame "Preset:LoadPreset" {
        # "Aggiorna il preset attuale\n(Tutte le volte che un preset viene modificato utilizzare questa funzione per aggiornare l'xml del preset attivo)"
        n189 = String To Path(string=w559) -> (path=w557:path)
        n190 = call "Preset_XML.vi"("SettingDataXmlPath"=w557, "error IO"=w555, "Actions"=enum16{"Init", "Read", "Write"}."Read") -> ("error out"=w554:errorcluster, "Preset Out"=w553:T9)  [unwired: 7 in]
        n191 = Bundle By Name(cluster=w552, "PresentPreset"=w553) -> (w551:T7)
        n192 = call <vilib>:"Add State(s) to Queue__JKI_lib_State_Machine.vi"("State(s) in (\"\")"=w561, "State(s) at Back (\"\")"="Preset:UpdatePresentPreset" ("State(s) at Back (\"\")")) -> ("States Out"=w560:string)  [unwired: 13 in]
      }
      frame "Preset: NewFile" {
        # "Create a New Preset File\n(Questo stato viene chiamato dal SetupList.vi e crea un nuovo file xml di setup)\n(Richiama il subpanel EditSetup con il parametro new o edit)"
        n193 = To Variant(anything=w564) -> (Variant=w563:variant)
        n194 = To Variant(anything="New") -> (Variant=w566:variant)
        n195 = Build Array(w566, w563) -> (w567:variant[])
        n196 = Build Array("Mode", "Setup#") -> (w569:string[])
        n197 = call <vilib>:"Build State String with Arguments__JKI_lib_State_Machine.vi"("Arguments (\"\")"="SetupEdit.vi" ("Arguments (\"\")"), "State"="SubPanel: Load" ("State(s) in Front (\"\")")) -> ("State with Arguments"=w571:string)  [unwired: 4 in]
        n198 = Bundle By Name(cluster=w574, "Control Names"=w569, "Values"=w567) -> (w570:T7)
        n199 = call <vilib>:"Add State(s) to Queue__JKI_lib_State_Machine.vi"("State(s) in Front (\"\")"=w571, "State(s) in (\"\")"=w577) -> ("States Out"=w576:string)  [unwired: 13 in]
      }
      frame "Preset: EditFile" {
        # "Edit Preset File\n(Questo stato viene chiamato dal SetupList.vi e richiama un  file xml di setup)\n(Richiama il subpanel EditSetup con il parametro new o edit)"
        n200 = String To Path(string=w584) -> (path=w579:path)
        n201 = Strip Path(path=w579) -> (name=w578:string)  [unwired: 1 out]
        n202 = call "Preset_UnflatFileName.vi"("error in (no error)"=w586, "PresetNameFile"=w578) -> ("error out"=w585:errorcluster, "Setup#"=w583:string, "Description"=w582:string)  [unwired: 6 in, 1 out]
        n203 = To Variant(anything="Edit") -> (Variant=w590:variant)
        n204 = To Variant(anything=w584) -> (Variant=w588:variant)
        n205 = To Variant(anything=w583) -> (Variant=w581:variant)
        n206 = To Variant(anything=w582) -> (Variant=w580:variant)
        n207 = Build Array(w590, w588, w581, w580) -> (w591:variant[])
        n208 = call <vilib>:"Build State String with Arguments__JKI_lib_State_Machine.vi"("Arguments (\"\")"="SetupEdit.vi" ("Arguments (\"\")"), "State"="SubPanel: Load" ("State(s) in Front (\"\")")) -> ("State with Arguments"=w593:string)  [unwired: 4 in]
        n209 = Bundle By Name(cluster=w596, "Control Names"=string[] ["Mode", "PresetFilePath", "Setup#", "Description"], "Values"=w591) -> (w592:T7)
        n210 = call <vilib>:"Add State(s) to Queue__JKI_lib_State_Machine.vi"("State(s) in Front (\"\")"=w593, "State(s) in (\"\")"=w598) -> ("States Out"=w597:string)  [unwired: 13 in]
      }
      frame "------------HW--------------" {
        # "HW SECTION\n(It is a separator no-op. You can make a copy of this frame to create a new UI frame)\n(You can make a copy of, or modify, this frame)"
        n211 = call <vilib>:"Add State(s) to Queue__JKI_lib_State_Machine.vi"("State(s) in (\"\")"=w602) -> ("States Out"=w601:string)  [unwired: 14 in]
      }
      frame "HW:SafeState" {
        # "HW SafeState\n(Qui posso mettere tutte le impoostazioni per il safe state)"
        n212 = disable-structure shown="Enabled" {
          disable-tunnel: w605 -> [w612 _]
          disable-tunnel: w604 -> [w610 _]
          disable-tunnel: [w609 _] -> w603
          frame Disabled {
            n213 = call-poly "Enqueue Message.vi"("error in (no error)"=w610, "Message"="SafeState", "Message Queue"=w612) -> ("error out"=w609:errorcluster)  [unwired: 7 in, 1 out]
          }
          frame Enabled {
            n214 = One Button Dialog(message="VAdo in safemode") -> ()  [unwired: 1 in, 1 out]
          }
        }
        n215 = call <vilib>:"Add State(s) to Queue__JKI_lib_State_Machine.vi"("State(s) in (\"\")"=w608) -> ("States Out"=w607:string)  [unwired: 14 in]
      }
      frame "HW:StandBy" {
        # "HW StandBY\n(Qui posso mettere tutte le impoostazioni per lo standBY)"
        n216 = disable-structure shown="Enabled" {
          disable-tunnel: w616 -> [w623 _]
          disable-tunnel: w615 -> [w621 _]
          disable-tunnel: [w620 _] -> w614
          frame Disabled {
            n217 = call-poly "Enqueue Message.vi"("error in (no error)"=w621, "Message"="SafeState", "Message Queue"=w623) -> ("error out"=w620:errorcluster)  [unwired: 7 in, 1 out]
          }
          frame Enabled {
            n218 = One Button Dialog(message="StandBy") -> ()  [unwired: 1 in, 1 out]
          }
        }
        n219 = call <vilib>:"Add State(s) to Queue__JKI_lib_State_Machine.vi"("State(s) in (\"\")"=w619) -> ("States Out"=w618:string)  [unwired: 14 in]
      }
      frame "HW:ReadyToPrint" {
        # "HW Ready To Print\n(La macchina è pronta a stampare e si mette in modalità ready to Print)\n(appena riceve il consenso dalla fotocellula inizia a stampare)"
        n220 = disable-structure shown="Disabled" {
          disable-tunnel: w627 -> [w634 _]
          disable-tunnel: w626 -> [w632 _]
          disable-tunnel: [w631 _] -> w625
          frame Disabled {
            n221 = call-poly "Enqueue Message.vi"("error in (no error)"=w632, "Message"="ReadyToPrint", "Message Queue"=w634) -> ("error out"=w631:errorcluster)  [unwired: 7 in, 1 out]
          }
          frame Enabled {
            n222 = One Button Dialog(message="StandBy") -> ()  [unwired: 1 in, 1 out]
          }
        }
        n223 = call <vilib>:"Add State(s) to Queue__JKI_lib_State_Machine.vi"("State(s) in (\"\")"=w630) -> ("States Out"=w629:string)  [unwired: 14 in]
      }
      frame "HW:InsertMatrix" {
        # "HW SafeState\n(Qui posso mettere tutte le impoostazioni per il safe state)"
        n224 = disable-structure shown="Disabled" {
          disable-tunnel: w639 -> [w647 _]
          disable-tunnel: w638 -> [w645 w648]
          disable-tunnel: [w644 w648] -> w637
          disable-tunnel: u64[] [] ("Buffer_U64") -> [w643 _]
          frame Disabled {
            n225 = call-poly "Enqueue Message.vi"("error in (no error)"=w645, "Message Data"=w643, "Message"="InsertMatrix", "Message Queue"=w647) -> ("error out"=w644:errorcluster)  [unwired: 6 in, 1 out]
          }
          frame Enabled {
            n226 = One Button Dialog(message="INSERT MATRIX") -> ()  [unwired: 1 in, 1 out]
          }
        }
        n227 = call <vilib>:"Add State(s) to Queue__JKI_lib_State_Machine.vi"("State(s) in (\"\")"=w642) -> ("States Out"=w641:string)  [unwired: 14 in]
      }
      frame "--------Login-----------" {
        # "LOGIN SECTION\n(It is a separator no-op. You can make a copy of this frame to create a new UI frame)\n(You can make a copy of, or modify, this frame)"
        n228 = call <vilib>:"Add State(s) to Queue__JKI_lib_State_Machine.vi"("State(s) in (\"\")"=w653) -> ("States Out"=w652:string)  [unwired: 14 in]
      }
      frame "Login:Fail" {
        # "LOGIN SECTION\n(It is a separator no-op. You can make a copy of this frame to create a new UI frame)\n(You can make a copy of, or modify, this frame)"
        n229 = One Button Dialog(message=w654) -> ()  [unwired: 1 in, 1 out]
        n230 = call <vilib>:"Add State(s) to Queue__JKI_lib_State_Machine.vi"("State(s) in (\"\")"=w655, "State(s) at Back (\"\")"="MainMenu:Login" ("State(s) at Back (\"\")")) -> ("States Out"=w659:string)  [unwired: 13 in]
      }
      frame "Login:Pass" {
        # "LOGIN SECTION\n(It is a separator no-op. You can make a copy of this frame to create a new UI frame)\n(You can make a copy of, or modify, this frame)"
        n231 = Spreadsheet String To Array(delimiter (Tab)=";", format string="", spreadsheet string=w670, array type (2D Dbl)=string[] []) -> (array=w669:string[])
        n232 = Index Array(array=w669) -> (element #1=w668:string, element #2=w667:string, element #3=w666:string)  [unwired: 3 in]
        n233 = Bundle By Name(cluster=T3 {"UsrName"="", "UsrPsw"="", "UsrLevel"=""} ("User"), "UsrName"=w668, "UsrPsw"=w667, "UsrLevel"=w666) -> (w664:T3)
        n234 = Bundle By Name(cluster=w663, "User"=w664) -> (w660:T7)
        n235 = Unbundle By Name(w660) -> ("User.UsrName"=w662:string)
        n236 = Format Into String(format string="\nWelcome %s", initial string=w661, w662) -> (resulting string=w675:string)  [unwired: 1 in, 1 out]
        n237 = One Button Dialog(message=w675) -> ()  [unwired: 1 in, 1 out]
        n238 = call <vilib>:"Add State(s) to Queue__JKI_lib_State_Machine.vi"("State(s) in (\"\")"=w676, "State(s) at Back (\"\")"="MainMenu: Main" ("State(s) at Back (\"\")")) -> ("States Out"=w679:string)  [unwired: 13 in]
      }
    }
  }
